vi "COD主界面（列队使用）.vi"() -> (8 "多列列表框":i32(listbox))   [LabVIEW 2016, in "斯坦道CODMn.lvlib"]
uses:
  <vilib>/Utility/miscctls.llb/LVPointTypeDef.ctl
  <vilib>/ptbypt/NI_PtbyPt.lvlib
  <vilib>/Utility/config.llb/NI_LVConfig.lvlib
panel:
  in  "温度补偿":bool
  in  "周期设置":bool
  out "F5":dbl
  out "F4":dbl
  out "F3":dbl
  out "F2":dbl
  out "F1":dbl
  out "F0":dbl
  out "消解压力kPa":dbl format="%#.2f"
  out "权限等级":string
  in  "布尔":bool
  in  "查看曲线":bool
  out "氢氧化钠":dbl
  in  "序列号变更":bool
  out "模块版本号":string
  in  "更新程序":bool
  out "进样无液体告警":bool
  out "60分钟超时报警":bool
  in  "仪器参数":bool
  in  "释放串口":bool
  in  "打开串口":bool
  out "报警数字":i16
  out "CODMn工作状态":T1(ring)
  out "ORP-K":string
  out "ORP-B":string
  out "ORP-A":string
  out "基本量程(显示)":string
  out "测量模式(显示)":string
  out "数据时间":string
  out "断电排液标记":bool
  out "COM":string
  out "空白测试标记":bool
  out "跨度核查标记":bool
  in  "手动控制":bool
  out "启动时间":timestamp format="%<%Y/%m/%d %H:%M:%S>T"
  out "零点核查标记":bool
  out "排液故障":bool
  out "进水样超量程":bool
  out "标样核查标记":bool
  out "平行样测量":bool
  out "加标回收测量":bool
  out "质控样测量":bool
  out "待机":bool
  out "校标错误":bool
  out "校零错误":bool
  out "测量错误":bool
  out "草酸钠报警":bool
  out "高锰酸钾报警":bool
  out "加热故障":bool
  out "温控器故障":bool
  out "ORP故障":bool
  out "排液标记":bool
  out "故障标记":bool
  out "校标标记":bool
  out "校零标记":bool
  out "通讯状态":bool
  out "水样测量":bool
  in  "返回":bool
  in  "校准配置":bool
  out "标度滴定值":dbl
  out "零点滴定值":dbl
  in  "保存":bool
  in  "关闭":bool
  out "仪器时间":timestamp format="%<%Y/%m/%d %H:%M:%S>T"
  out "秒":u16
  out "分":u16
  out "COD浓度（mg/L)":dbl format="%.2g"
  out "进样管":dbl
  out "高锰酸钾":dbl
  out "草酸钠":dbl
  out "硫酸":dbl
  out "实时ORP/光值":dbl
  out "消解温度℃":dbl
  out "加热":bool
  out "搅拌":bool
  out "进硫酸":bool
  out "进加标回收样":bool
  out "进零点核查样":bool
  out "进标液":bool
  out "进蒸馏水":bool
  out "进水样":bool
  out "进草酸钠":bool
  out "进高锰酸钾":bool
  in  "启动":bool
  in  "故障清除":bool
  in  "参数配置":bool
  in  "停止":bool
  in  "单步启动":bool
  out "系统时间":timestamp
  in  "时间校准":bool
  out "模式（受控）":u16
  # "测试时长："
  # "注：遇到加热故障和排液故障时仪器不能正常启动，\n必须排查故障并点击报警清除按钮方可运行。"
  # "mg/L"
  # "校零校标结果"
  # "校零结果："
  # "校零滴定值："
  # "校标结果："
  # "标度滴定值："
  # "零点泵计量值："
  # "标度泵计量值："
  # "校准配置界面"
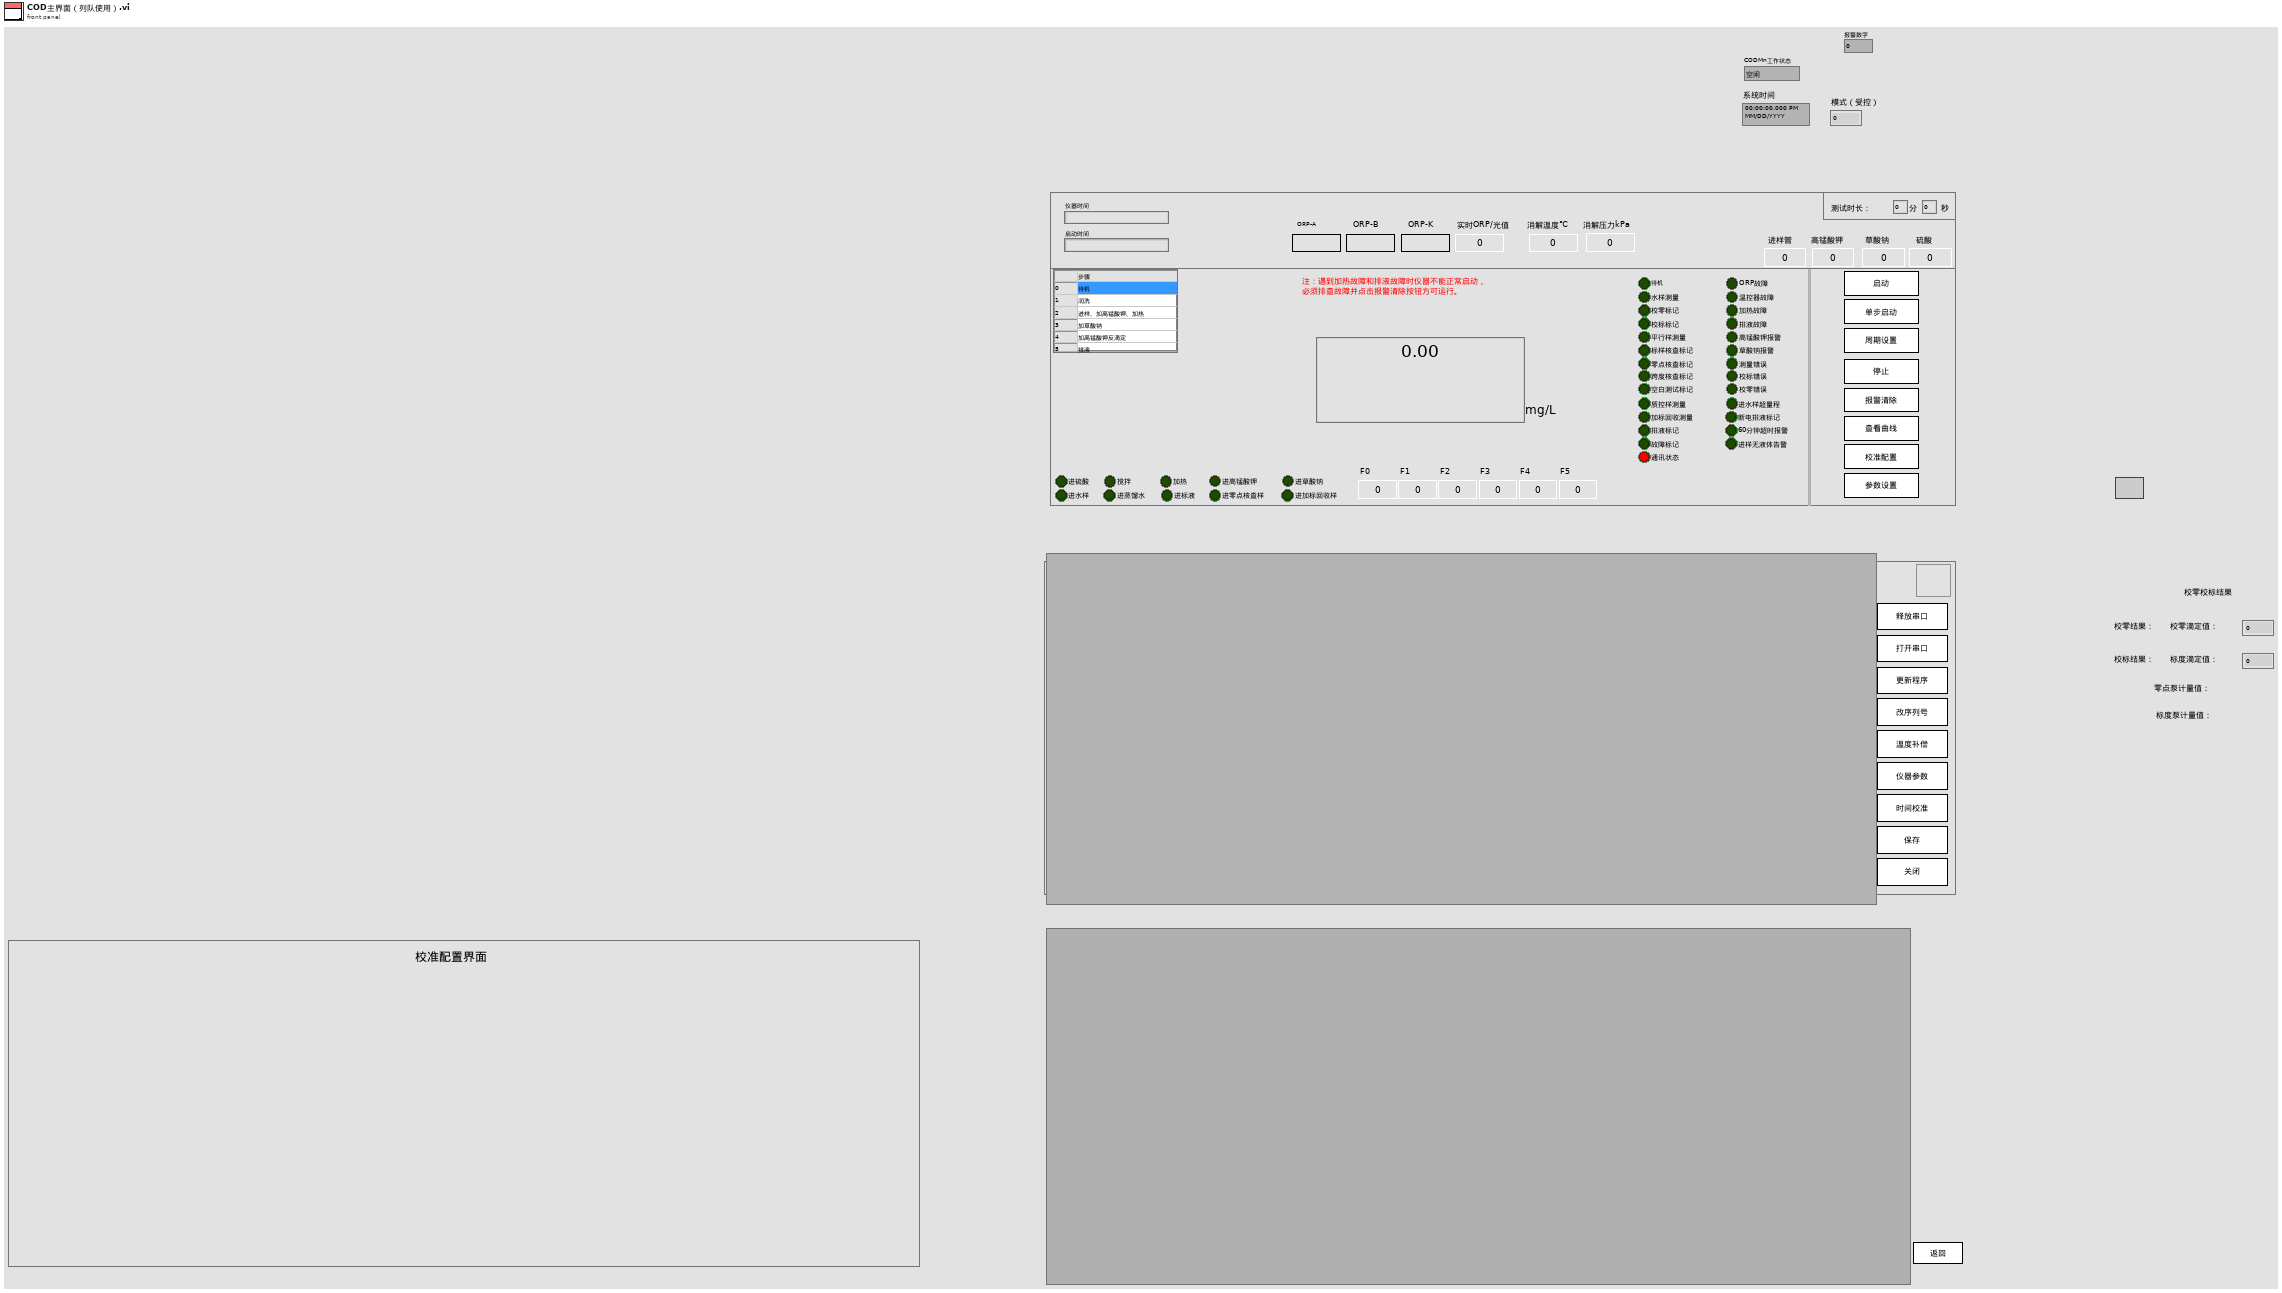
[diagram p1: front panel]
types:
  T1 = enum16{"空闲", "水样测试", "标样核查", "零点核查", "跨度核查", "空白测试", "平行样测试", "质控样", "空白校准", "标样校准", "加标回收"}
  T2 = typedef "LVPointTypeDef.ctl" = cluster{"Horizontal":i16, "Vertical":i16}
  T3 = cluster{"Major":u16, "Minor":u16, "Fix":u16, "Build":u16}
  T4 = typedef "NI_LVConfig.lvlib/Config Data RefNum.ctl" = refnum<k1>
  T5 = cluster{"运行模式":enum16{"维护模式", "常规模式", "应急模式", "质控模式"}, "质控频次":enum16{"关闭", "每天", "星期一", "星期二", "星期三", "星期四", "星期五", "星期六", "星期日"}, "空白核查时间":u16, "跨度核查时间":u16, "测量间隔":u16}
  T6 = cluster{"测量量程":dbl, "测量精度":dbl, "测量间隔":dbl, "消解温度":dbl, "消解时长":dbl, "空白校准时间":timestamp, "曲线截距":dbl, "曲线斜率":dbl, "测量检出限":dbl, "测量信号值":dbl, "线性相关系数":dbl, "二次多项式系数":dbl, "标样校准时间":timestamp, "稀释倍数":dbl, "三项式系数":dbl, "空白标定系数":dbl, "量程系数":dbl, "F0/ORPA":dbl, "F1/ORPB":dbl, "F2/ORPK":dbl, "F3":dbl, "F4":dbl, "F5":dbl, "F6":dbl, "F7":dbl, "X0/滴定数":dbl, "量程":dbl}
  T7 = typedef "TimingControl.lvlib/TimingControl.lvclass/国标控制命令.ctl" = enum16{"启动测量", "标样核查", "零点核查", "跨度核查", "空白测试", "平行样测试", "加标回收", "空白校准", "标样校准", "初始化（清洗）", "停止测试", "仪器重启", "校时", "模式设置", "测量间隔设置"}
  T8 = typedef "TimingControl.lvlib/TimingControl.lvclass/测量参数.ctl" = u16
  T9 = enum32{"Bad", "Idle", "Run top level", "Running"}
  T10 = enum8{"Enabled", "Disabled", "Disabled and Grayed Out"}
  T11 = cluster{"因子编码":u32, "单位":u16, "标样参考值":sgl, "水样数据时间":timestamp, "水样实测值":sgl, "水样数据标识":string, "标样数据时间":timestamp, "标样实测值":sgl, "标样数据标识":string, "空白数据时间":timestamp, "空白实测值":sgl, "空白数据标识":string, "零点核查数据时间":timestamp, "零点核查实测值":sgl, "零点核查数据标识":string, "跨度核查数据时间":timestamp, "跨度核查实测值":sgl, "跨度核查数据标识":string, "加标回收数据时间":timestamp, "加标回收实测值":sgl, "加标回收数据标识":string, "平行样数据时间":timestamp, "平行样实测值":sgl, "平行样数据标识":string}
  T12 = cluster{"时间":timestamp, "测量模式":string, "数据类型":string, "检测值":sgl, "单位":string, "数据标识":string, "因子编码":string, "标样参考值":sgl, "ORP-A":sgl, "ORP-B":sgl, "ORP-K":sgl, "COD滴定值":sgl, "高锰酸钾滴定数":sgl, "温度":sgl, "量程":sgl, "LastTime":timestamp, "序列号:":string, "跨度值":sgl, "高锰酸钾原始滴定数":sgl, "F0":sgl, "F1":sgl, "F2":sgl, "F3":sgl, "F4":sgl, "F5":sgl}
  T13 = cluster{"ORP故障":bool, "温控器故障":bool, "加热故障":bool, "高锰酸钾报警":bool, "草酸钠报警":bool, "测量错误":bool, "校零错误":bool, "校标错误":bool, " 进水样超量程":bool, "排液阀故障":bool, "60分钟超时报警":bool, "进样无液体报警":bool}
  T14 = cluster{"时间":timestamp, "水样计量数":u16, "蒸馏水计量数":u16, "标液计量数":u16, "零点核查计量数":u16, "加标回收计量数":u16, "硫酸计量数":u16, "高锰酸钾计量数":u16, "草酸钠计量数":u16, "更换泵管":string}
  T15 = cluster{"确定":bool, "测量量程":dbl, "测量精度":dbl, "测量间隔":dbl, "消解温度":dbl, "消解时长":dbl, "空白校准时间":timestamp, "曲线截距":dbl, "曲线斜率":dbl, "测量检出限":dbl, "测量信号值":dbl, "线性相关系数":dbl, "二次多项式系数":dbl, "标样校准时间":timestamp, "稀释倍数":dbl, "三项式系数":dbl, "空白标定系数":dbl, "量程系数":dbl, "F0/ORPA":dbl, "F1/ORPB":dbl, "F2/ORPK":dbl, "F3":dbl, "F4":dbl, "F5":dbl, "F6":dbl, "F7":dbl, "X0/滴定数":dbl, "量程":dbl}
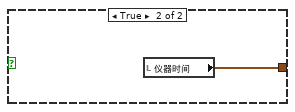
[diagram p6: hidden frame]
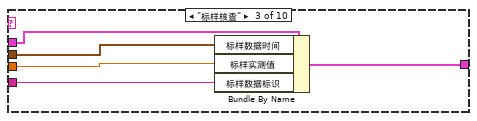
[diagram p13: hidden frame]
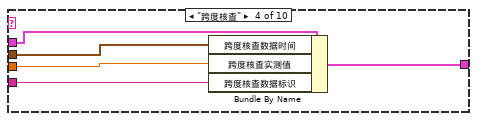
[diagram p14: hidden frame]
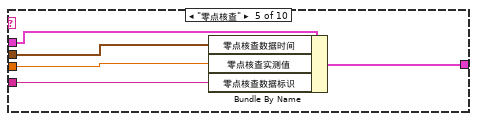
[diagram p15: hidden frame]
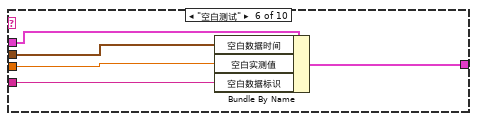
[diagram p16: hidden frame]
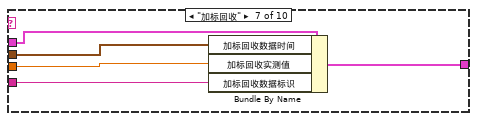
[diagram p17: hidden frame]
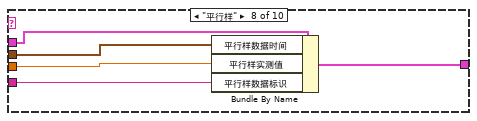
[diagram p18: hidden frame]
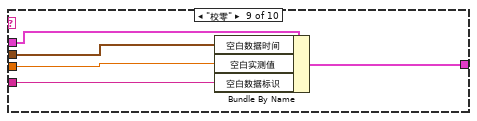
[diagram p19: hidden frame]
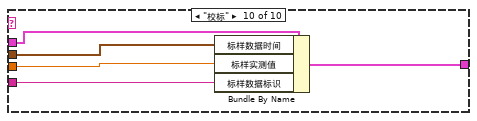
[diagram p20: hidden frame]
diagram:
  n1 = control-ref of="周期设置"() -> (w5:refnum<vi>)
  n2 = call "New TimingControl.vi"("Reference"=w5) -> ("error out"=w3:errorcluster, "TimingControl out"=w4:refnum<class "TimingControl.lvclass">)  [unwired: 9 in]
  n3 = call "taskqueue ref.vi"() -> ("队列输出"=w16:refnum<queue>)  [unwired: 10 in, 1 out]
  n4 = call "task.vi"() -> ()  [unwired: 12 in]
  n5 = flat-sequence {
    tunnel: [w33] -> w19
    tunnel: [errorcluster {"status"=FALSE, "code"=0, "source"=""} ("错误输出")] -> w17
    tunnel: [w35] -> w18
    frame #0 {
      w57 = "192.168.1.100" ("名称")
      n6 = global read "COD内部交互全局.vi" "序列号:"() -> (w64:string)
      n7 = global write "COD内部交互全局.vi" "量程切换次数"(u8 0 ("量程切换次数")) -> ()
      n8 = global write "COD内部交互全局.vi" "切换量程连续测两次"(FALSE ("切换量程连续测两次")) -> ()
      n9 = property on="窗格" class="Pane"("Origin"=T2 {"Horizontal"=0, "Vertical"=0} ("原点")) -> ()  [unwired: 2 in, 2 out]
      n10 = control-ref of="本VI"() -> (w44:refnum<vi>)
      n11 = property class="VI"(reference=w44) -> ("Library.Version"=w43:T3)  [unwired: 1 in, 2 out]
      n12 = Empty String/Path?(string/path=w64) -> (empty?=w32:bool)
      n13 = case shown="真" w32 {
        tunnel: w64 -> [w76 _]
        tunnel: [w75 "data\\CODMnSet.ini" ("名称或相对路径")] -> w45
        frame False {
          # "与生产用上位机交互"
          n14 = Concatenate Strings("data\\" ("字符串"), "序列号" ("字符串"), w76, "Set.ini" ("名称或相对路径")) -> (w75:string)
        }
        frame True {
        }
      }
      n15 = Unbundle By Name(w43) -> ("Major"=w41:u16, "Minor"=w40:u16, "Fix"=w39:u16, "Build"=w38:u16)
      n16 = String To IP(1:w57) -> (0:w50:u32)
      n17 = Format Into String(format string="模块版本号：%d.%d.%d.%d" ("格式字符串"), w41, w40, w39, w38) -> (resulting string=→"模块版本号":string)  [unwired: 2 in, 1 out]
      n18 = IP To String(2:w50) -> (0:w53:string)  [unwired: 1 in]
      n19 = Not Equal?(x=w57, y=w53) -> (x != y?=w58:bool)
      n20 = Concatenate Strings("\\\\" ("字符串"), w53) -> (w52:string)
      n21 = global write "CODMN外部API.vi" "ping"(w58) -> ()
      n22 = String To Path(string=w52) -> (path=w59:path)
      n23 = global write "COD内部交互全局.vi" "配置文件ini"(w45) -> ()
      n24 = Build Path(base path=w59, name or relative path=w45) -> (appended path=w54:path)
      n25 = case shown="真" w58 {
        tunnel: w54 -> [w66 w70]
        tunnel: [w66 w69] -> w55
        tunnel: [FALSE w68] -> w56
        frame False {
        }
        frame True {
          n26 = call <vilib>:"Check if File or Folder Exists.vi"("path"=w70) -> ("file or folder exists?"=w68:bool, "dup path"=w69:path)  [unwired: 8 in, 1 out]
        }
      }
      n27 = case shown="假" w56 {
        tunnel: w55 -> [_ w74]
        tunnel: [w72 w74] -> w36
        tunnel: w45 -> [w71 _]
        frame False {
          # "本地文件地址"
          n28 = call <vilib>:"Application Directory.vi"() -> ("Application Directory"=w73:path)
          n29 = Build Path(base path=w73, name or relative path=w71) -> (appended path=w72:path)
        }
        frame True {
          # "网络共享地址"
        }
      }
      n30 = global write "CODMN外部API.vi" "配置文件 path"(w36) -> ()
      n31 = call <vilib>:"Open Config Data.vi"("configuration file path"=w36) -> ("error out"=w46:errorcluster, "refnum"=w47:T4)  [unwired: 8 in, 1 out]
      n32 = vi-ref "斯坦道CODMn.lvlib:CODMn断电保存全局变量.vi"() -> (w60:refnum<vi>)
      n33 = call <userlib>:"Read Panel from INI__ogtk.vi"("error in (no error)"=w46, "VI ref"=w60, "refnum"=w47) -> ("error out"=w48:errorcluster, "refnum out"=w49:T4)  [unwired: 7 in]
      n34 = call <vilib>:"Close Config Data.vi"("error in (no error)"=w48, "refnum"=w49) -> ("error out"=w34:errorcluster)  [unwired: 8 in, 1 out]
      n35 = call <vilib>:"Clear Errors.vi"("error in (no error)"=w34) -> ("error out"=w31:errorcluster)  [unwired: 5 in, 1 out]
      n36 = Read from Text File(file (use dialog)=w36, error in=w31) -> (text=w35:string, error out=w33:errorcluster)  [unwired: 2 in, 2 out]
    }
  }
  n37 = while {
    stop <- FALSE stop-if-true
    # "相差60秒自动校时"
    n38 = global read "运行时序全局变量.vi" "多列列表框"() -> (w84:i32)
    n39 = local read "消解温度℃"() -> (w81:dbl)
    n40 = local read "仪器时间"() -> (w91:timestamp)
    n41 = local read "系统时间"() -> (w92:timestamp)
    n42 = Wait (ms)(milliseconds to wait=u32 1000 ("等待时间（毫秒）")) -> ()  [unwired: 1 out]
    n43 = call "消解压力计算.vi"("当前消解温度"=w81) -> ("消解压力"=→"消解压力kPa":dbl)  [unwired: 10 in]
    n44 = Build Array(w91) -> (w90:timestamp[])
    n45 = Build Array(w92) -> (w109:timestamp[])
    n46 = Equal?(x=w84, y=u16 5) -> (x = y?=w86:bool)
    n47 = call <vilib>:"Boolean Crossing PtByPt.vi"("direction"=enum16{"either", "false-true", "true-false"}."false-true", "input"=w86) -> ("crossing"=w83:bool)  [unwired: 1 in]
    n48 = call "DateToHex.vi"("DATE"=w90) -> ("数组"=w103:u16[])  [unwired: 10 in]
    n49 = call "DateToHex.vi"("DATE"=w109) -> ("数组"=w108:u16[])  [unwired: 10 in]
    n50 = case shown="真" w83 {
      frame False {
      }
      frame True {
        # "校准结束后自动更新曲线泵滴定数"
        n51 = global read "CODMN外部API.vi" "远程反控校准CODMn"() -> (w110:bool)
        n52 = case shown="真" w110 {
          frame False {
          }
          frame True {
            # "校准完自动写入公式"
            n53 = global write "CODMN外部API.vi" "远程反控校准CODMn"(FALSE ("远程反控校准CODMn")) -> ()
          }
        }
      }
    }
    n54 = Index Array(array=w103, index=2 ("索引")) -> (element=w105:u16)
    n55 = Index Array(array=w108, index=2 ("索引")) -> (element=w106:u16)
    n56 = Split Number(x=w105) -> (hi(x)=w99:u8)  [unwired: 1 out]
    n57 = Split Number(x=w106) -> (hi(x)=w102:u8)  [unwired: 1 out]
    n58 = To Byte Integer(number=w99) -> (8bit integer=w98:i8)
    n59 = To Byte Integer(number=w102) -> (8bit integer=w101:i8)
    n60 = Subtract(x=w98, y=w101) -> (x-y=w100:i8)
    n61 = Absolute Value(x=w100) -> (abs(x)=w97:i8)
    n62 = local read "通讯状态"() -> (w94:bool)
    n63 = Greater Or Equal?(x=w97, y=i8 5) -> (x >= y?=w95:bool)
    n64 = And(x=w95, y=w94) -> (x .and. y?=w93:bool)
    n65 = case shown="真" w93 {
      frame False {
      }
      frame True {
        # "相差60秒时间自动校准"
        n66 = flat-sequence {
          frame #0 {
            n67 = property on="时间校准" class="Bool (严格)"("Val(Sgnl)"=TRUE ("值(信号)")) -> ()  [unwired: 2 in, 2 out]
          }
          frame #1 {
            n68 = Wait (ms)(milliseconds to wait=u32 500 ("等待时间（毫秒）")) -> ()  [unwired: 1 out]
          }
          frame #2 {
            n69 = property on="时间校准" class="Bool (严格)"("Val(Sgnl)"=FALSE ("值(信号)")) -> ()  [unwired: 2 in, 2 out]
          }
        }
      }
    }
  }
  n70 = while {
    tunnel: w16 -> [w133]
    shift-right: [w125] -> _
    shift-left: 0 -> [w124]
    shift-right: [w116] -> w2
    shift-left: w4 -> [w121]
    shift-right: [w115] -> w1
    shift-left: w3 -> [w120]
    stop <- FALSE stop-if-true
    n71 = global read "CODMn断电保存全局变量.vi" "运行周期"() -> (w135:T5)
    n72 = local read "通讯状态"() -> (w138:bool)
    n73 = Quotient & Remainder(x=w124, y=30) -> (x-y*floor(x/y)=w122:i32)  [unwired: 1 out]
    n74 = Equal To 0?(x=w122) -> (x = 0?=w129:bool)
    n75 = global read "CODMn断电保存全局变量.vi" "CODMn仪器参数"() -> (w137:T6)
    n76 = Unbundle By Name(w135) -> ("测量间隔"=w134:u16)
    n77 = case shown="假" w138 {
      tunnel: [w149 w150] -> w118
      frame False {
        n78 = Get Date/Time In Seconds() -> (seconds since 1Jan1904=w149:timestamp)
      }
      frame True {
        n79 = local read "仪器时间"() -> (w150:timestamp)
      }
    }
    n80 = Bundle By Name(cluster=w137, "测量间隔"=w134) -> (w136:T6)
    n81 = global read "COD测量模式全局.vi" "CODMn工作状态"() -> (w130:T1)
    n82 = Not Equal?(x=w130, y=T1."空闲") -> (x != y?=w117:bool)
    n83 = global write "CODMn断电保存全局变量.vi" "CODMn仪器参数"(w136) -> ()
    n84 = property class="TimingControl"(reference=w121, error in=w120, "Properties:仪器时间"=w118, "Properties:仪器运行状态"=w117) -> (reference out=w116:refnum<class "TimingControl.lvclass">, error out=w115:errorcluster, "Properties:命令输出"=w119:cluster{"启动":bool, "控制命令":T7, "测量参数":T8})
    n85 = Increment(x=w124) -> (x+1=w127:i32)
    n86 = Unbundle By Name(w119) -> ("启动"=w128:bool, "控制命令"=w132:T7)
    n87 = And(x=w128, y=w129) -> (x .and. y?=w131:bool)
    n88 = Select(t=w127, s=w128, f=0) -> (s? t:f=w125:i32)
    n89 = case shown="真" w131 {
      tunnel: w133 -> [_ w146]
      tunnel: w132 -> [_ w145]
      frame False {
      }
      frame True {
        n90 = Get Queue Status(queue=w146) -> (queue out=w144:refnum<queue>, # elements in queue=w143:i32)  [unwired: 2 in, 6 out]
        n91 = Equal To 0?(x=w143) -> (x = 0?=w142:bool)
        n92 = case shown="真" w142 {
          tunnel: w145 -> [_ w148]
          tunnel: w144 -> [_ w147]
          frame False {
          }
          frame True {
            n93 = Enqueue Element(queue=w147, element=w148) -> ()  [unwired: 2 in, 3 out]
          }
        }
      }
    }
    n94 = Wait (ms)(milliseconds to wait=u32 500 ("等待时间（毫秒）")) -> ()  [unwired: 1 out]
  }
  n95 = vi-ref "斯坦道CODMn.lvlib:参数设置页.vi"() -> (w7:refnum<vi>)
  n96 = vi-ref "校准设置页.vi"() -> (w14:refnum<vi>)
  n97 = property class="VI"(reference=w7) -> (reference out=w9:refnum<vi>, "Exec.State"=w8:T9)  [unwired: 1 in, 1 out]
  n98 = property class="VI"(reference=w14) -> (reference out=w12:refnum<vi>, "Exec.State"=w13:T9)  [unwired: 1 in, 1 out]
  n99 = case shown="\"Idle\"" w8 {
    tunnel: w9 -> [w151 w155]
    tunnel: [w151 w152] -> w6
    frame "Bad", Default {
    }
    frame "Idle" {
      n100 = invoke class="VI" method="Run VI"(reference=w155, "Wait until done"=FALSE ("结束前等待"), "Auto Dispose Ref"=TRUE ("自动销毁引用")) -> (reference out=w152:refnum<vi>)  [unwired: 2 in, 4 out]
    }
  }
  n101 = case shown="\"Idle\"" w13 {
    tunnel: w12 -> [w156 w160]
    tunnel: [w156 w157] -> w11
    frame "Bad", Default {
    }
    frame "Idle" {
      n102 = invoke class="VI" method="Run VI"(reference=w160, "Wait until done"=FALSE ("结束前等待"), "Auto Dispose Ref"=TRUE ("自动销毁引用")) -> (reference out=w157:refnum<vi>)  [unwired: 2 in, 4 out]
    }
  }
  n103 = call "Close TimingControl.vi"("error in (no error)"=w1, "TimingControl in"=w2) -> ()  [unwired: 9 in, 1 out]
  n104 = Obtain Queue(name (unnamed)="CODMn", element data type=cluster{"命令":string} {"命令"="启用模块"} ("元素")) -> (queue out=w29:refnum<queue>, error out=w28:errorcluster)  [unwired: 3 in, 1 out]
  n105 = while {
    tunnel: w19 -> [_]
    stop <- FALSE stop-if-true
    # "赋值循环"
    n106 = flat-sequence {
      frame #0 {
        # "局部变量给内部交互用全局变量"
        n107 = local read "待机"() -> (w168:bool)
        n108 = local read "实时ORP/光值"() -> (w163:dbl)
        n109 = local read "消解温度℃"() -> (w164:dbl)
        n110 = local read "多列列表框"() -> (w170:i32)
        n111 = local read "故障标记"() -> (w171:bool)
        n112 = local read "高锰酸钾"() -> (w165:dbl)
        n113 = global write "COD内部交互全局.vi" "待机"(w168) -> ()
        n114 = local read "COD浓度（mg/L)"() -> (w169:dbl)
        n115 = local read "CODMn工作状态"() -> (w172:T1)
        n116 = local read "断电排液标记"() -> (w166:bool)
        n117 = local read "高锰酸钾报警"() -> (w167:bool)
        n118 = global write "COD内部交互全局.vi" "故障标记"(w171) -> ()
        n119 = global write "COD内部交互全局.vi" "ORP显示"(w163) -> ()
        n120 = global write "COD内部交互全局.vi" "高锰酸钾"(w165) -> ()
        n121 = global write "COD内部交互全局.vi" "实时温度"(w164) -> ()
        n122 = global write "运行时序全局变量.vi" "多列列表框"(w170) -> ()
        n123 = global write "COD浓度全局变量.vi" "COD浓度（mg/L)"(w169) -> ()
        n124 = global write "COD内部交互全局.vi" "断电排液标记"(w166) -> ()
        n125 = global write "COD内部交互全局.vi" "高锰酸钾报警"(w167) -> ()
        n126 = global write "COD测量模式全局.vi" "CODMn工作状态"(w172) -> ()
      }
    }
    n127 = flat-sequence {
      frame #0 {
        # "断电保存全局给局部变量"
        n128 = global read "CODMn断电保存全局变量.vi" "启动时间"() -> (→"启动时间":timestamp)
      }
    }
    n129 = flat-sequence {
      frame #0 {
        # "显示量程说明"
        n130 = global read "COD内部交互全局.vi" "通讯状态"() -> (→"通讯状态":bool)
        n131 = global read "CODMn断电保存全局变量.vi" "MB通信方式选择"() -> (w238:enum16{"串口", "TCP"})
        n132 = case shown="\"TCP\"" w238 {
          tunnel: [w241 w242] -> w240
          frame "串口", Default {
            n133 = global read "CODMn断电保存全局变量.vi" "VISA resource name"() -> (w241:refnum<visa-resource-name>)
          }
          frame "TCP" {
            n134 = global read "CODMn断电保存全局变量.vi" "IP"() -> (w242:string)
          }
        }
        "COM" <- w240
      }
    }
    n135 = flat-sequence {
      frame #0 {
        # "权限隐藏和显示功能"
        n136 = global read "CODMN外部API.vi" "权限等级"() -> (w248:enum16{"一级权限", "二级权限", "三级权限", "超级权限"})
        n137 = global read "CODMn断电保存全局变量.vi" "常规版/认证版"() -> (w244:enum16{"常规版-酸性", "常规版-碱性", "认证版", "浮台版"})
        n138 = case shown="\"二级权限\"" w248 {
          tunnel: [w253 FALSE w258 w260] -> w245
          tunnel: ["一级权限" "二级权限" "三级权限" "超级权限"] -> w247
          tunnel: [w253 TRUE w258 w260] -> w246
          frame "一级权限", Default {
            w253 = FALSE
          }
          frame "二级权限" {
          }
          frame "三级权限" {
            w258 = TRUE
          }
          frame "超级权限" {
            w260 = TRUE
          }
        }
        "权限等级" <- w247
        n139 = global read "CODMn断电保存全局变量.vi" "CODMn系统周期测试?"() -> (w249:bool)
        n140 = case shown="\"浮台版\"" w244 {
          tunnel: [T10."Enabled" ("禁用") T10."Enabled" ("禁用") T10."Disabled and Grayed Out" ("禁用") T10."Enabled" ("禁用")] -> _
          tunnel: [i32[] [2] ("禁用项[]") i32[] [2] ("禁用项[]") i32[] [] ("禁用项[]") i32[] [2] ("禁用项[]")] -> _
          tunnel: [w271 w276 T10."Disabled and Grayed Out" ("禁用") w287] -> _
          tunnel: [w270 FALSE FALSE TRUE] -> _
          tunnel: [w271 w276 T10."Disabled and Grayed Out" ("禁用") w287] -> w252
          tunnel: [w270 TRUE FALSE FALSE] -> w251
          frame "常规版-酸性", Default {
            w270 = FALSE
            w271 = T10."Enabled" ("禁用")
          }
          frame "常规版-碱性" {
            w276 = T10."Enabled" ("禁用")
          }
          frame "认证版" {
            w282 = u16 1 items=["水样测试"=1, "标样核查"=2, "零点核查"=3, "跨度核查"=4, "空白测试"=5, "平行样"=6, "加标回收"=7] ("测量模式(公式)")
            n141 = global write "CODMn断电保存全局变量.vi" "测量模式(公式)"(w282) -> ()
          }
          frame "浮台版" {
            w287 = T10."Enabled" ("禁用")
          }
        }
        n142 = global read "CODMn断电保存全局变量.vi" "运行周期"() -> (w250:T5)
        n143 = case shown="真" w249 {
          tunnel: w250 -> [_ w265]
          tunnel: [T10."Enabled" ("禁用") w263] -> _
          frame False {
          }
          frame True {
            n144 = Unbundle By Name(w265) -> ("运行模式"=w264:enum16{"维护模式", "常规模式", "应急模式", "质控模式"})
            n145 = case shown="\"维护模式\", 默认" w264 {
              tunnel: [T10."Enabled" ("禁用") T10."Disabled and Grayed Out" ("禁用") T10."Disabled and Grayed Out" ("禁用") T10."Disabled and Grayed Out" ("禁用")] -> w263
              frame "维护模式", Default {
              }
              frame "常规模式" {
              }
              frame "应急模式" {
              }
              frame "质控模式" {
              }
            }
          }
        }
        n146 = property on="更新程序" class="Bool (严格)"("Visible"=w245) -> ()  [unwired: 2 in, 2 out]
        n147 = property on="释放串口" class="Bool"("Visible"=w246) -> ()  [unwired: 2 in, 2 out]
        n148 = property on="打开串口" class="Bool"("Visible"=w246) -> ()  [unwired: 2 in, 2 out]
        n149 = property on="序列号变更" class="Bool"("Visible"=w245) -> ()  [unwired: 2 in, 2 out]
        n150 = property on="氢氧化钠" class="DigNum (严格)"("Visible"=w251) -> ()  [unwired: 2 in, 2 out]
        n151 = control-ref of="进样管"() -> (w243:refnum<vi>)
        n152 = property class="DigNum (严格)"(reference=w243, "DisabledEnum"=w252) -> ()  [unwired: 1 in, 2 out]
      }
    }
    n153 = flat-sequence {
      frame #0 {
        # "测量数据区"
        n154 = global read "CODMn断电保存全局变量.vi" "测量数据区"() -> (w185:T11)
        n155 = global read "COD内部交互全局.vi" "data"() -> (w190:T12)
        n156 = global read "COD测量模式全局.vi" "测量模式文字实时"() -> (w176:string)
        "测量模式(显示)" <- w176
        n157 = global read "CODMn断电保存全局变量.vi" "水样测试量程"() -> (w178:enum16{"L", "H"})
        n158 = Unbundle By Name(w185) -> ("水样实测值"=w182:sgl)
        n159 = global read "CODMn断电保存全局变量.vi" "测量模式"() -> (w174:string)
        n160 = Unbundle By Name(w190) -> ("时间"=w189:timestamp, "检测值"=w188:sgl, "数据标识"=w187:string)
        n161 = feedback-in #1(w185) -> ()
        n162 = feedback #1(w185) -> (w184:T11)
        n163 = Unbundle By Name(w184) -> ("水样实测值"=w183:sgl)
        n164 = case shown="\"水样测试\"" w176 {
          tunnel: w185 -> [w191 w196 w201 w206 w211 w216 w221 w226 w231 w236]
          tunnel: [w191 w195 w200 w202 w210 w215 w220 w225 w227 w235] -> w186
          tunnel: w189 -> [_ w194 w199 w205 w209 w214 w219 w224 w230 w234]
          tunnel: w188 -> [_ w193 w198 w204 w208 w213 w218 w223 w229 w233]
          tunnel: w187 -> [_ w192 w197 w203 w207 w212 w217 w222 w228 w232]
          frame "", Default {
          }
          frame "水样测试" {
            n165 = Bundle By Name(cluster=w196, "水样数据时间"=w194, "水样实测值"=w193, "水样数据标识"=w192) -> (w195:T11)
          }
          frame "标样核查" {
            n166 = Bundle By Name(cluster=w201, "标样数据时间"=w199, "标样实测值"=w198, "标样数据标识"=w197) -> (w200:T11)
          }
          frame "跨度核查" {
            n167 = Bundle By Name(cluster=w206, "跨度核查数据时间"=w205, "跨度核查实测值"=w204, "跨度核查数据标识"=w203) -> (w202:T11)
          }
          frame "零点核查" {
            n168 = Bundle By Name(cluster=w211, "零点核查数据时间"=w209, "零点核查实测值"=w208, "零点核查数据标识"=w207) -> (w210:T11)
          }
          frame "空白测试" {
            n169 = Bundle By Name(cluster=w216, "空白数据时间"=w214, "空白实测值"=w213, "空白数据标识"=w212) -> (w215:T11)
          }
          frame "加标回收" {
            n170 = Bundle By Name(cluster=w221, "加标回收数据时间"=w219, "加标回收实测值"=w218, "加标回收数据标识"=w217) -> (w220:T11)
          }
          frame "平行样" {
            n171 = Bundle By Name(cluster=w226, "平行样数据时间"=w224, "平行样实测值"=w223, "平行样数据标识"=w222) -> (w225:T11)
          }
          frame "校零" {
            n172 = Bundle By Name(cluster=w231, "空白数据时间"=w230, "空白实测值"=w229, "空白数据标识"=w228) -> (w227:T11)
          }
          frame "校标" {
            n173 = Bundle By Name(cluster=w236, "标样数据时间"=w234, "标样实测值"=w233, "标样数据标识"=w232) -> (w235:T11)
          }
        }
        n174 = feedback #2(w178) -> (w179:enum16{"L", "H"})
        n175 = feedback-in #2(w178) -> ()
        n176 = feedback #3(w174) -> (w175:string)
        n177 = feedback-in #3(w174) -> ()
        n178 = Not Equal?(x=w175, y=w174) -> (x != y?=w173:bool)
        n179 = Not Equal?(x=w179, y=w178) -> (x != y?=w177:bool)
        n180 = Not Equal?(x=w182, y=w183) -> (x != y?=w181:bool)
        n181 = Compound Arithmetic op=OR ("复合运算")(w181, w177, w173) -> (w180:bool)
        n182 = case shown="真" w180 {
          frame False {
          }
          frame True {
            # "水样值发送改变存储本地"
            n183 = call "配置文件保存.vi"() -> ()  [unwired: 12 in]
          }
        }
        n184 = global write "CODMn断电保存全局变量.vi" "测量数据区"(w186) -> ()
      }
    }
    n185 = Wait (ms)(milliseconds to wait=u32 1000 ("等待时间（毫秒）")) -> ()  [unwired: 1 out]
  }
  n186 = while {
    tunnel: [w297] -> _
    shift-right: [w295] -> _
    shift-left: w18 -> [w294]
    tunnel: w19 -> [_]
    stop <- FALSE stop-if-true
    n187 = Wait (ms)(milliseconds to wait=u32 1000 ("等待时间（毫秒）")) -> ()  [unwired: 1 out]
    n188 = global read "CODMN外部API.vi" "配置文件 path"() -> (w291:path)
    n189 = Read from Text File(file (use dialog)=w291) -> (text=w295:string, error out=w292:errorcluster)  [unwired: 3 in, 2 out]
    n190 = Not Equal?(x=w295, y=w294) -> (x != y?=w293:bool)
    n191 = case shown="真" w293 {
      tunnel: [w299 w306] -> w297
      tunnel: w291 -> [_ w300]
      tunnel: w292 -> [w299 _]
      frame False {
      }
      frame True {
        # "文件发生改变进行更新，远端和本地都更新"
        n192 = call <vilib>:"Open Config Data.vi"("configuration file path"=w300) -> ("error out"=w305:errorcluster, "refnum"=w304:T4)  [unwired: 8 in, 1 out]
        n193 = vi-ref "斯坦道CODMn.lvlib:CODMn断电保存全局变量.vi"() -> (w301:refnum<vi>)
        n194 = call <userlib>:"Read Panel from INI__ogtk.vi"("error in (no error)"=w305, "VI ref"=w301, "refnum"=w304) -> ("error out"=w303:errorcluster, "refnum out"=w302:T4)  [unwired: 7 in]
        n195 = call <vilib>:"Close Config Data.vi"("error in (no error)"=w303, "refnum"=w302) -> ("error out"=w306:errorcluster)  [unwired: 8 in, 1 out]
      }
    }
  }
  n196 = flat-sequence {
    tunnel: w17 -> [_]
    frame #0 {
      n197 = vi-ref "斯坦道CODMn.lvlib:关键参数交互.vi"() -> (w324:refnum<vi>)
      n198 = vi-ref "斯坦道CODMn.lvlib:时间-温度曲线(子VI).vi"() -> (w315:refnum<vi>)
      n199 = property class="VI"(reference=w324, error in=errorcluster {"status"=FALSE, "code"=0, "source"=""} ("错误输出")) -> ("Name"=w323:string)  [unwired: 2 out]
      n200 = vi-ref "斯坦道CODMn.lvlib:高锰酸钾-ORP滴定曲线(子VI).vi"() -> (w333:refnum<vi>)
      n201 = vi-ref "斯坦道CODMn.lvlib:日志报警状态存储 (子VI).vi"() -> (w346:refnum<vi>)
      n202 = vi-ref "斯坦道CODMn.lvlib:待机状态数据存储写入和切换量程(子VI).vi"() -> (w353:refnum<vi>)
      n203 = property class="VI"(reference=w315, error in=errorcluster {"status"=FALSE, "code"=0, "source"=""} ("错误输出")) -> ("Name"=w314:string)  [unwired: 2 out]
      n204 = property class="VI"(reference=w346, error in=errorcluster {"status"=FALSE, "code"=0, "source"=""} ("错误输出")) -> ("Name"=w345:string)  [unwired: 2 out]
      n205 = property class="VI"(reference=w333, error in=errorcluster {"status"=FALSE, "code"=0, "source"=""} ("错误输出")) -> ("Name"=w334:string)  [unwired: 2 out]
      n206 = Open VI Reference(type specifier VI Refnum (for type only)=refnum<vi> refnum, vi path=w323, options=128 ("选项")) -> (vi reference=w325:refnum<vi>, error out=w321:errorcluster)  [unwired: 3 in]
      n207 = property class="VI"(reference=w353, error in=errorcluster {"status"=FALSE, "code"=0, "source"=""} ("错误输出")) -> ("Name"=w352:string)  [unwired: 2 out]
      n208 = Open VI Reference(type specifier VI Refnum (for type only)=refnum<vi> refnum, vi path=w314, options=128 ("选项")) -> (vi reference=w316:refnum<vi>, error out=w312:errorcluster)  [unwired: 3 in]
      n209 = Open VI Reference(type specifier VI Refnum (for type only)=refnum<vi> refnum, vi path=w345, options=128 ("选项")) -> (vi reference=w329:refnum<vi>, error out=w343:errorcluster)  [unwired: 3 in]
      n210 = Open VI Reference(type specifier VI Refnum (for type only)=refnum<vi> refnum, vi path=w334, options=128 ("选项")) -> (vi reference=w332:refnum<vi>, error out=w336:errorcluster)  [unwired: 3 in]
      n211 = call-by-ref "?"(reference=w316, error in=w312) -> (reference out=w310:refnum<vi>, error out=w311:errorcluster)  [unwired: 12 in]
      n212 = call-by-ref "?"(reference=w325, error in=w321, "量程选择"=enum16{"低量程", "高量程"}."低量程", "模型"=enum32{"线性", "多项式", "折线"}."线性") -> (reference out=w319:refnum<vi>, error out=w320:errorcluster)  [unwired: 10 in]
      n213 = Close Reference(reference=w310, error in (no error)=w311) -> ()  [unwired: 1 out]
      n214 = Close Reference(reference=w319, error in (no error)=w320) -> ()  [unwired: 1 out]
      n215 = call-by-ref "?"(reference=w329, error in=w343) -> (reference out=w341:refnum<vi>, error out=w342:errorcluster)  [unwired: 12 in]
      n216 = call-by-ref "?"(reference=w332, error in=w336) -> (reference out=w338:refnum<vi>, error out=w337:errorcluster)  [unwired: 12 in]
      n217 = Open VI Reference(type specifier VI Refnum (for type only)=refnum<vi> refnum, vi path=w352, options=128 ("选项")) -> (vi reference=w327:refnum<vi>, error out=w350:errorcluster)  [unwired: 3 in]
      n218 = Close Reference(reference=w341, error in (no error)=w342) -> ()  [unwired: 1 out]
      n219 = Close Reference(reference=w338, error in (no error)=w337) -> ()  [unwired: 1 out]
      n220 = call-by-ref "?"(reference=w327, error in=w350) -> (reference out=w348:refnum<vi>, error out=w349:errorcluster)  [unwired: 12 in]
      n221 = Close Reference(reference=w348, error in (no error)=w349) -> ()  [unwired: 1 out]
    }
  }
  n222 = vi-ref "CODMn通讯.vi"() -> (w20:refnum<vi>)
  n223 = while {
    tunnel: w29 -> [w363]
    tunnel: w28 -> [w362]
    tunnel: w19 -> [_]
    stop <- FALSE stop-if-true
    # "主循环界面显示"
    n224 = flat-sequence {
      frame #0 {
        # "A，B，K"
        # "CODMn读取状态"
        n225 = global read "COD内部交互全局.vi" "ORP、时间"() -> (w510:u16[])
        n226 = To Word Integer(number=w510) -> (16bit integer=w528:i16[])
        n227 = Split 1D Array(array=w528, index=3 ("索引")) -> (first subarray=w512:i16[], second subarray=w527:i16[])
        n228 = global read "CODMn断电保存全局变量.vi" "屏蔽负值"() -> (w508:bool)
        n229 = Index Array(array=w512) -> (element #1=w516:i16, element #2=w515:i16, element #3=w514:i16)  [unwired: 3 in]
        n230 = Index Array(array=w527) -> (element #1=w507:i16, element #2=w526:i16, element #3=w525:i16, element #4=w524:i16)  [unwired: 4 in]
        n231 = case shown="真" w508 {
          selector: w508 -> [w530 _]
          tunnel: w507 -> [w532 w537]
          tunnel: [w531 w540] -> w506
          tunnel: [w530 w536] -> _
          frame False {
            n232 = To Single Precision Float(number=w532) -> (single precision float=w534:sgl)
            n233 = Divide(x=w534, y=sgl 100.0) -> (x/y=w531:sgl)
          }
          frame True {
            n234 = To Single Precision Float(number=w537) -> (single precision float=w538:sgl)
            n235 = Divide(x=w538, y=sgl 100.0) -> (x/y=w535:sgl)
            n236 = Less Or Equal To 0?(x=w535) -> (x <= 0?=w536:bool)
            n237 = case shown="真" w536 {
              tunnel: [w541 sgl 0.015] -> w540
              tunnel: w535 -> [w541 _]
              frame False {
              }
              frame True {
              }
            }
          }
        }
        "COD浓度（mg/L)" <- w506
        n238 = To Single Precision Float(number=w524) -> (single precision float=w518:sgl)
        n239 = Build Array(w516, w515, w514) -> (w513:i16[])
        n240 = To Single Precision Float(number=w526) -> (single precision float=w523:sgl)
        n241 = To Single Precision Float(number=w525) -> (single precision float=w519:sgl)
        n242 = call "HexToDate.vi"("数组"=w513) -> ("DATE"=w517:timestamp[])  [unwired: 10 in]
        n243 = Number To Decimal String(number=w523) -> (decimal integer string=→"ORP-A":string)  [unwired: 1 in]
        n244 = Number To Decimal String(number=w519) -> (decimal integer string=→"ORP-B":string)  [unwired: 1 in]
        n245 = Number To Decimal String(number=w518) -> (decimal integer string=→"ORP-K":string)  [unwired: 1 in]
        n246 = Index Array(array=w517) -> (element=w511:timestamp)  [unwired: 1 in]
        n247 = Format Date/Time String(seconds (now)=w511) -> (date/time string=→"数据时间":string)  [unwired: 2 in]
      }
    }
    n248 = flat-sequence {
      frame #0 {
        # "测量状态显示"
        n249 = global read "COD内部交互全局.vi" "F0-F5"() -> (w414:u16[])
        n250 = global read "COD内部交互全局.vi" "测量状态"() -> (w422:u16[])
        n251 = To Single Precision Float(number=w414) -> (single precision float=w413:sgl[])
        n252 = Index Array(array=w413) -> (element #1=→"F0":sgl, element #2=→"F1":sgl, element #3=→"F2":sgl, element #4=→"F3":sgl, element #5=→"F4":sgl, element #6=→"F5":sgl)  [unwired: 6 in]
        n253 = To Word Integer(number=w422) -> (16bit integer=w432:i16[])
        n254 = Index Array(array=w432, index #1=0 ("索引"), index #4=3 ("索引"), index #14=13 ("索引"), index #15=14 ("索引"), index #21=20 ("索引"), index #32=31 ("索引")) -> (element #1=w436:i16, element #2=w435:i16, element #3=w434:i16, element #4=w418:i16, element #5=→"模式（受控）":i16, element #6=→"进样管":i16, element #7=→"高锰酸钾":i16, element #8=→"草酸钠":i16, element #9=→"硫酸":i16, element #10=w431:i16, element #11=w451:i16, element #12=w427:i16, element #13=→"报警数字":i16, element #14=w457:i16, element #15=w442:i16, element #16=→"多列列表框":i16, element #20=→"氢氧化钠":i16, element #21=w415:i16, element #33=→"分":i16, element #34=→"秒":i16)  [unwired: 28 in, 14 out]
        "CODMn工作状态" <- w418
        n255 = global write "COD内部交互全局.vi" "基本量程实时读取"(w415) -> ()
        n256 = Equal?(x=w418, y=T1."水样测试" ("CODMn工作状态")) -> (x = y?=w416:bool)
        n257 = Build Array(w436, w435, w434) -> (w437:i16[])
        n258 = To Single Precision Float(number=w431) -> (single precision float=→"实时ORP/光值":sgl)
        n259 = Number To Decimal String(number=w415) -> (decimal integer string=→"基本量程(显示)":string)  [unwired: 1 in]
        n260 = Equal?(x=w427, y=u16 1) -> (x = y?=→"排液标记":bool)
        n261 = Equal?(x=w427, y=u16 2) -> (x = y?=→"断电排液标记":bool)
        n262 = Divide(x=w451, y=u16 10) -> (x/y=→"消解温度℃":dbl)
        n263 = Divide(x=w457, y=u16 1000) -> (x/y=→"零点滴定值":dbl)
        n264 = Divide(x=w442, y=u16 1000) -> (x/y=→"标度滴定值":dbl)
        n265 = case shown="真" w416 {
          tunnel: w415 -> [_ w460]
          frame False {
          }
          frame True {
            n266 = global write "CODMn断电保存全局变量.vi" "水样测试量程"(w460) -> ()
          }
        }
        n267 = call "HexToDate.vi"("数组"=w437) -> ("DATE"=w433:timestamp[])  [unwired: 10 in]
        n268 = Index Array(array=w433) -> (element=→"仪器时间":timestamp)  [unwired: 1 in]
      }
    }
    n269 = flat-sequence {
      frame #0 {
        # "报警状态显示"
        n270 = global read "COD内部交互全局.vi" "报警点位"() -> (w475:bool[])
        n271 = Index Array(array=w475, index #1=0 ("索引")) -> (element #1=w472:bool, element #2=w471:bool, element #3=w470:bool, element #4=w469:bool, element #5=w468:bool, element #6=w467:bool, element #7=w466:bool, element #8=w465:bool, element #9=w464:bool, element #11=w463:bool, element #13=w462:bool, element #14=w461:bool)  [unwired: 13 in, 2 out]
        "ORP故障" <- w472
        "温控器故障" <- w471
        "加热故障" <- w464
        "高锰酸钾报警" <- w466
        "草酸钠报警" <- w465
        "测量错误" <- w470
        "校零错误" <- w469
        "校标错误" <- w468
        "进水样超量程" <- w467
        "排液故障" <- w463
        "60分钟超时报警" <- w462
        "进样无液体告警" <- w461
        n272 = Compound Arithmetic op=OR ("复合运算")(w472, w471, w464, w466, w465, w470, w468, w469, w467, w463, w462) -> (→"故障标记":bool)
        n273 = Bundle By Name(cluster=T13 {"ORP故障"=FALSE, "温控器故障"=FALSE, "加热故障"=FALSE, "高锰酸钾报警"=FALSE, "草酸钠报警"=FALSE, "测量错误"=FALSE, "校零错误"=FALSE, "校标错误"=FALSE, " 进水样超量程"=FALSE, "排液阀故障"=FALSE, "60分钟超时报警"=FALSE, "进样无液体报警"=FALSE} ("报警簇"), "ORP故障"=w472, "温控器故障"=w471, "加热故障"=w464, "高锰酸钾报警"=w466, "草酸钠报警"=w465, "测量错误"=w470, "校零错误"=w469, "校标错误"=w468, "进水样超量程"=w467, "排液阀故障"=w463, "60分钟超时报警"=w462, "进样无液体报警"=w461) -> (w473:T13)
        n274 = global write "COD内部交互全局.vi" "报警簇"(w473) -> ()
      }
    }
    n275 = flat-sequence {
      frame #0 {
        # "CODMn读取状态"
        n276 = global read "COD内部交互全局.vi" "温度"() -> (w505:bool[])
        n277 = global read "COD内部交互全局.vi" "M输出点"() -> (w504:bool[])
        n278 = Index Array(array=w505) -> (element=→"加热":bool)  [unwired: 1 in]
        n279 = Index Array(array=w504) -> (element #1=→"搅拌":bool, element #4=→"进水样":bool, element #5=→"进蒸馏水":bool, element #6=→"进标液":bool, element #7=→"进零点核查样":bool, element #8=→"进加标回收样":bool, element #9=→"进高锰酸钾":bool, element #10=→"进草酸钠":bool, element #11=→"进硫酸":bool)  [unwired: 11 in, 2 out]
      }
    }
    n280 = flat-sequence {
      frame #0 {
        # "工作状态显示"
        n281 = local read "CODMn工作状态"() -> (w373:T1)
        n282 = Not Equal To 0?(x=w373) -> (x != 0?=w372:bool)
        n283 = Equal?(x=w373, y=u16 0) -> (x = y?=→"待机":bool)
        n284 = Equal?(x=w373, y=u16 8) -> (x = y?=→"校零标记":bool)
        n285 = Equal?(x=w373, y=u16 1) -> (x = y?=→"水样测量":bool)
        n286 = Equal?(x=w373, y=u16 9) -> (x = y?=→"校标标记":bool)
        n287 = Equal?(x=w373, y=u16 7) -> (x = y?=→"质控样测量":bool)
        n288 = Equal?(x=w373, y=u16 5) -> (x = y?=→"空白测试标记":bool)
        n289 = Equal?(x=w373, y=u16 4) -> (x = y?=→"跨度核查标记":bool)
        n290 = Equal?(x=w373, y=u16 3) -> (x = y?=→"零点核查标记":bool)
        n291 = Equal?(x=w373, y=u16 2) -> (x = y?=→"标样核查标记":bool)
        n292 = Equal?(x=w373, y=u16 6) -> (x = y?=→"平行样测量":bool)
        n293 = Equal?(x=w373, y=u16 10) -> (x = y?=→"加标回收测量":bool)
        n294 = case shown="真" w372 {
          tunnel: w373 -> [_ w397]
          frame False {
          }
          frame True {
            n295 = case shown="\"水样测试\"" w397 {
              tunnel: [_ u16 0 ("y") u16 1 ("y") u16 2 ("y") u16 3 ("y") u16 4 ("y") u16 6 ("y") _ u16 7 ("y") u16 8 ("y") u16 5 ("y")] -> w396
              frame "空闲", Default {
              }
              frame "水样测试" {
              }
              frame "标样核查" {
              }
              frame "零点核查" {
              }
              frame "跨度核查" {
              }
              frame "空白测试" {
              }
              frame "平行样测试" {
              }
              frame "质控样" {
              }
              frame "空白校准" {
              }
              frame "标样校准" {
              }
              frame "加标回收" {
              }
            }
            n296 = global write "COD内部交互全局.vi" "测量模式数字"(w396) -> ()
          }
        }
      }
    }
    n297 = Get Date/Time In Seconds() -> (seconds since 1Jan1904=→"系统时间":timestamp)
    n298 = First Call?() -> (First Call?: T/F=w361:bool)
    n299 = Wait (ms)(milliseconds to wait=u32 1000 ("等待时间（毫秒）")) -> ()  [unwired: 1 out]
    n300 = case shown="真" w361 {
      tunnel: w363 -> [w479 w490]
      tunnel: w362 -> [w478 w489]
      tunnel: [w479 w481] -> w359
      tunnel: [w478 w480] -> w358
      frame False {
      }
      frame True {
        n301 = Bundle By Name(cluster=cluster{"命令":string} {"命令"=""} ("元素"), "命令"="CODMn读取参数" ("名称（未命名）")) -> (w493:cluster{"命令":string})
        n302 = Bundle By Name(cluster=cluster{"命令":string} {"命令"=""} ("元素"), "命令"="CODMn读取公式" ("名称（未命名）")) -> (w484:cluster{"命令":string})
        n303 = Enqueue Element(queue=w490, element=w493, timeout in ms (-1)=1000 ("超时毫秒(-1)"), error in (no error)=w489) -> (queue out=w483:refnum<queue>, error out=w482:errorcluster)  [unwired: 1 out]
        n304 = Enqueue Element(queue=w483, element=w484, timeout in ms (-1)=1000 ("超时毫秒(-1)"), error in (no error)=w482) -> (queue out=w481:refnum<queue>, error out=w480:errorcluster)  [unwired: 1 out]
      }
    }
    n305 = Get Queue Status(queue=w359, error in (no error)=w358) -> (queue out=w355:refnum<queue>, error out=w354:errorcluster, # elements in queue=w357:i32)  [unwired: 1 in, 5 out]
    n306 = Equal To 0?(x=w357) -> (x = 0?=w356:bool)
    n307 = case shown="真" w356 {
      tunnel: w355 -> [_ w367]
      tunnel: w354 -> [_ w366]
      frame False {
      }
      frame True {
        n308 = Bundle By Name(cluster=cluster{"命令":string} {"命令"=""} ("元素"), "命令"="CODMn读取" ("名称（未命名）")) -> (w369:cluster{"命令":string})
        n309 = Enqueue Element(queue=w367, element=w369, timeout in ms (-1)=1000 ("超时毫秒(-1)"), error in (no error)=w366) -> ()  [unwired: 3 out]
      }
    }
  }
  n310 = while {
    tunnel: w29 -> [w546]
    tunnel: w28 -> [w545]
    tunnel: w11 -> [w544]
    tunnel: w6 -> [w543]
    stop <- FALSE stop-if-true
    # "主线事件"
    n311 = event shown="[19] \"温度补偿\": 值改变" {
      selector: _ -> [_ _ _ _ _ _ _ _ _ _ _ _ _ _ _ _ _ _ _ _ _]
      dyn-events: _ -> [_ _ _ _ _ _ _ _ _ _ _ _ _ _ _ _ _ _ _ _ _]
      timeout: _ -> [_ _ _ _ _ _ _ _ _ _ _ _ _ _ _ _ _ _ _ _ _]
      tunnel: w546 -> [_ _ _ _ w625 _ _ w668 _ _ _ _ _ _ _ w723 w730 w752 w796 w813 _]
      tunnel: w545 -> [_ _ _ _ w624 _ _ w667 _ _ _ _ _ _ _ w722 w729 w751 w795 w812 _]
      tunnel: w544 -> [_ _ _ _ _ _ _ w666 _ _ _ _ _ _ _ _ _ _ _ _ _]
      tunnel: w543 -> [_ _ _ _ w620 _ _ _ _ _ _ _ _ _ _ _ _ _ _ _ _]
      event "单步启动": Value Change {
        n312 = event-data() -> ()  [unwired: 1 in, 6 out]
        n313 = call "CODMn手动控制框.vi"() -> ()  [unwired: 12 in]
      }
      event "启动": Mouse Down {
        n314 = event-data() -> ()  [unwired: 1 in, 8 out]
        n315 = global read "COD内部交互全局.vi" "基本量程实时读取"() -> (w550:enum16{"L", "H", "AUTO"})
        n316 = call "启动测量模式选择对话框.vi"("量程选择"=w550) -> ("标样浓度输出"=w548:dbl, "量程选择输出"=w549:enum16{"L", "H", "AUTO"}, "启动选择输出"=w554:u16)  [unwired: 8 in]
        n317 = Not Equal?(x=w554, y=u16 7) -> (x != y?=w552:bool)
        n318 = Not Equal?(x=w554, y=u16 8) -> (x != y?=w551:bool)
        n319 = And(x=w552, y=w551) -> (x .and. y?=w556:bool)
        n320 = case shown="真" w556 {
          tunnel: w554 -> [_ w571]
          tunnel: w549 -> [_ w562]
          tunnel: w548 -> [_ w561]
          frame False {
            n321 = One Button Dialog(message="请到校准配置里面进行校准操作！" ("消息")) -> ()  [unwired: 1 in, 1 out]
          }
          frame True {
            n322 = case shown="4" w571 {
              tunnel: [u16 4608 ("address") u16 4608 ("address") u16 4608 ("address") u16 4608 ("address") u16 4608 ("address") u16 4608 ("address") u16 4608 ("address") u16 4608 ("address") u16 4608 ("address") u16 4608 ("address")] -> w564
              tunnel: [u16 1 ("address") u16 2 ("address") u16 3 ("address") u16 4 ("address") u16 5 ("address") u16 7 ("address") u16 6 ("address") u16 8 ("address") u16 9 ("address") u16 0 ("address")] -> w568
              tunnel: w561 -> [_ _ _ _ _ _ _ _ _ _]
              frame 0 {
              }
              frame 1 {
              }
              frame 2 {
              }
              frame 3 {
              }
              frame 4 {
              }
              frame 5 {
              }
              frame 6 {
              }
              frame 7 {
              }
              frame 8 {
              }
              frame 9, Default {
              }
            }
            n323 = case shown="\"H\"" w562 {
              tunnel: [w572 w576 errorcluster {"status"=FALSE, "code"=0, "source"=""} ("error out")] -> w560
              frame "L", Default {
                n324 = call "CODMnMB_api.vi"("STEP"=enum16{"open", "read", "write", "close"}."write", "values"=u16[] [0], "starting address"=u16 4276) -> ("error out"=w572:errorcluster)  [unwired: 6 in, 2 out]
              }
              frame "H" {
                n325 = call "CODMnMB_api.vi"("STEP"=enum16{"open", "read", "write", "close"}."write", "values"=u16[] [1], "starting address"=u16 4276) -> ("error out"=w576:errorcluster)  [unwired: 6 in, 2 out]
              }
              frame "AUTO" {
              }
            }
            n326 = Not Equal?(x=w571, y=u16 9) -> (x != y?=w566:bool)
            n327 = global write "CODMN外部API.vi" "手动启动CODMn"(w566) -> ()
            n328 = call "单步测试一键复位.vi"("Error in"=w560) -> ("error out"=w559:errorcluster)  [unwired: 10 in]
            n329 = call <vilib>:"Clear Errors.vi"("error in (no error)"=w559) -> ("error out"=w558:errorcluster)  [unwired: 5 in, 1 out]
            n330 = Insert Into Array(array=u16[] [] ("values"), index=0 ("索引"), new element=w568) -> (w563:u16[])
            n331 = call "CODMnMB_api.vi"("STEP"=enum16{"open", "read", "write", "close"}."write", "Error in"=w558, "values"=w563, "starting address"=w564) -> ()  [unwired: 5 in, 3 out]
          }
        }
      }
      event "停止": Value Change {
        n332 = event-data() -> ()  [unwired: 1 in, 6 out]
        n333 = Two Button Dialog(message="确认是否停止？" ("消息"), 1:"否" ("F按钮名称（“取消”）"), 2:"是" ("T按钮名称（“确定”）")) -> (T button?=w603:bool)
        n334 = case shown="真" w603 {
          frame False {
          }
          frame True {
            n335 = Obtain Notifier(name (unnamed)="CODMn" ("名称（未命名）"), notification data type=FALSE) -> (notifier out=w609:refnum<notifier>, error out=w607:errorcluster)  [unwired: 2 in, 1 out]
            n336 = Send Notification(notification=TRUE ("通知"), notifier=w609, error in (no error)=w607) -> (notifier out=w606:refnum<notifier>, error out=w605:errorcluster)
            n337 = call "CODMnMB_api.vi"("STEP"=enum16{"open", "read", "write", "close"}."write", "values"=u16[] [11], "starting address"=u16 4608) -> ()  [unwired: 6 in, 3 out]
            n338 = Release Notifier(notifier=w606, error in (no error)=w605) -> ()  [unwired: 1 in, 3 out]
          }
        }
      }
      event "手动控制": Value Change {
        n339 = event-data() -> ()  [unwired: 1 in, 6 out]
        n340 = call "数字密码键盘.vi"() -> ("NewNumber"=w615:u32)  [unwired: 1 in]
        n341 = Equal?(x=w615, y=8.0) -> (x = y?=w616:bool)
        n342 = case shown="假" w616 {
          frame False {
            n343 = call "窗口弹出对话框(子VI).vi"("消息"="密码错误") -> ()  [unwired: 10 in, 1 out]
          }
          frame True {
          }
        }
      }
      event "参数配置": Value Change {
        (unwired) u16 20 ("number of holding registers")
        n344 = event-data() -> ()  [unwired: 1 in, 6 out]
        n345 = global read "CODMN外部API.vi" "ping"() -> (w623:bool)
        n346 = invoke on="子面板" class="SubPnl" method="Remove VI"() -> (error out=w619:errorcluster)  [unwired: 3 in, 2 out]
        n347 = property on="窗格" class="Pane"("Origin"=T2 {"Horizontal"=0, "Vertical"=650} ("原点")) -> ()  [unwired: 2 in, 2 out]
        n348 = case shown="假" w623 {
          tunnel: [w635 w638] -> w622
          frame False {
            n349 = global read "COD内部交互全局.vi" "配置文件ini"() -> (w637:string)
            n350 = call <vilib>:"Application Directory.vi"() -> ("Application Directory"=w636:path)
            n351 = Build Path(base path=w636, name or relative path=w637) -> (appended path=w635:path)
          }
          frame True {
            n352 = global read "CODMN外部API.vi" "配置文件 path"() -> (w638:path)
          }
        }
        n353 = invoke on="子面板" class="SubPnl" method="Insert VI"(error in=w619, "VI Ref"=w620) -> ()  [unwired: 2 in, 4 out]
        n354 = Bundle By Name(cluster=cluster{"命令":string} {"命令"=""} ("元素"), "命令"="CODMn读取参数" ("名称（未命名）")) -> (w626:cluster{"命令":string})
        n355 = Enqueue Element(queue=w625, element=w626, error in (no error)=w624) -> ()  [unwired: 1 in, 3 out]
        n356 = call <vilib>:"Open Config Data.vi"("configuration file path"=w622) -> ("error out"=w632:errorcluster, "refnum"=w629:T4)  [unwired: 8 in, 1 out]
        n357 = vi-ref "斯坦道CODMn.lvlib:CODMn断电保存全局变量.vi"() -> (w630:refnum<vi>)
        n358 = call <userlib>:"Read Panel from INI__ogtk.vi"("error in (no error)"=w632, "VI ref"=w630, "refnum"=w629) -> ("error out"=w633:errorcluster, "refnum out"=w631:T4)  [unwired: 7 in]
        n359 = call <vilib>:"Close Config Data.vi"("error in (no error)"=w633, "refnum"=w631) -> ("error out"=w621:errorcluster)  [unwired: 8 in, 1 out]
        n360 = call <vilib>:"Clear Errors.vi"("error in (no error)"=w621) -> ()  [unwired: 5 in, 2 out]
      }
      event "布尔": Value Change {
        n361 = event-data() -> ("CtlRef"=w639:refnum<vi>, "NewVal"=w640:bool)  [unwired: 1 in, 4 out]
        n362 = case shown="真" w640 {
          tunnel: w639 -> [_ w643]
          frame False {
            n363 = global write "CODMN外部API.vi" "权限等级"(enum16{"一级权限", "二级权限", "三级权限", "超级权限"}."一级权限" ("权限等级")) -> ()
          }
          frame True {
            n364 = property class="Bool (严格)"(reference=w643, "Value"=FALSE ("值")) -> ()  [unwired: 1 in, 2 out]
            n365 = global read "CODMN外部API.vi" "权限密码"() -> (w644:u32[])
            n366 = global read "CODMN外部API.vi" "权限等级"() -> (w646:enum16{"一级权限", "二级权限", "三级权限", "超级权限"})
            n367 = call "密码权限设置.vi"("权限输入"=w646, "权限密码"=w644) -> ("权限输出"=w645:enum16{"一级权限", "二级权限", "三级权限", "超级权限"})  [unwired: 9 in]
            n368 = global write "CODMN外部API.vi" "权限等级"(w645) -> ()
          }
        }
      }
      event "保存": Value Change {
        n369 = event-data() -> ()  [unwired: 1 in, 6 out]
        n370 = local read "通讯状态"() -> (w647:bool)
        n371 = Two Button Dialog(message="确定保存参数，保存参数将会替换原有参数！" ("消息")) -> (T button?=w649:bool)  [unwired: 2 in]
        n372 = case shown="真" w649 {
          tunnel: w647 -> [_ w650]
          frame False {
          }
          frame True {
            n373 = case shown="真" w650 {
              frame False {
                n374 = One Button Dialog(message="保存失败，当前无通讯！" ("消息")) -> ()  [unwired: 1 in, 1 out]
              }
              frame True {
                n375 = global read "COD内部交互全局.vi" "保存参数"() -> (w652:dbl[])
                n376 = One Button Dialog(message="参数保存成功！" ("消息")) -> ()  [unwired: 1 in, 1 out]
                n377 = global read "COD内部交互全局.vi" "采水泵参数"() -> (w653:i32[])
                n378 = call "CODMnMB_api.vi"("STEP"=enum16{"open", "read", "write", "close"}."write", "values"=w652, "starting address"=u16 4272) -> ("error out"=w660:errorcluster)  [unwired: 6 in, 2 out]
                n379 = call "CODMnMB_api.vi"("STEP"=enum16{"open", "read", "write", "close"}."write", "Error in"=w660, "values"=w653, "starting address"=u16 5596) -> ("error out"=w657:errorcluster)  [unwired: 5 in, 2 out]
                n380 = global read "COD内部交互全局.vi" "泵校准参数"() -> (w654:T14)
                n381 = call <vilib>:"Clear Errors.vi"("error in (no error)"=w657) -> ("error out"=w655:errorcluster)  [unwired: 5 in, 1 out]
                n382 = call "PLC版CODMn泵校准数据插入.vi"("data"=w654, "错误输入（无错误）"=w655) -> ("错误输出"=w656:errorcluster)  [unwired: 8 in]
                n383 = flat-sequence {
                  tunnel: w656 -> [_]
                  frame #0 {
                    n384 = global write "COD内部交互全局.vi" "更换泵管"(FALSE ("更换泵管")) -> ()
                  }
                }
              }
            }
          }
        }
      }
      event "校准配置": Value Change {
        n385 = event-data() -> ()  [unwired: 1 in, 6 out]
        n386 = invoke on="子面板" class="SubPnl" method="Remove VI"() -> (error out=w665:errorcluster)  [unwired: 3 in, 2 out]
        n387 = property on="窗格" class="Pane"("Origin"=T2 {"Horizontal"=0, "Vertical"=1300} ("原点")) -> ()  [unwired: 2 in, 2 out]
        n388 = invoke on="子面板" class="SubPnl" method="Insert VI"(error in=w665, "VI Ref"=w666) -> ()  [unwired: 2 in, 4 out]
        n389 = Bundle By Name(cluster=cluster{"命令":string} {"命令"=""} ("元素"), "命令"="CODMn读取公式" ("名称（未命名）")) -> (w669:cluster{"命令":string})
        n390 = Enqueue Element(queue=w668, element=w669, error in (no error)=w667) -> ()  [unwired: 1 in, 3 out]
      }
      event "返回": Value Change {
        n391 = event-data() -> ()  [unwired: 1 in, 6 out]
        n392 = property on="窗格" class="Pane"("Origin"=T2 {"Horizontal"=0, "Vertical"=0} ("原点")) -> ()  [unwired: 2 in, 2 out]
      }
      event "关闭": Value Change {
        n393 = event-data() -> ()  [unwired: 1 in, 6 out]
        n394 = property on="窗格" class="Pane"("Origin"=T2 {"Horizontal"=0, "Vertical"=0} ("原点")) -> ()  [unwired: 2 in, 2 out]
      }
      event Application Instance Close {
        n395 = event-data() -> ()  [unwired: 1 in, 4 out]
      }
      event "时间校准": Value Change {
        n396 = event-data() -> ()  [unwired: 1 in, 6 out]
        n397 = Get Date/Time In Seconds() -> (seconds since 1Jan1904=w683:timestamp)
        n398 = Build Array(w683) -> (w682:timestamp[])
        n399 = call "DateToHex.vi"("DATE"=w682) -> ("数组"=w680:u16[])  [unwired: 10 in]
        n400 = Insert Into Array(array=u16[] [1] ("values"), index=1 ("索引"), new element=w680) -> (w676:u16[])
        n401 = call "CODMnMB_api.vi"("STEP"=enum16{"open", "read", "write", "close"}."write", "values"=w676, "starting address"=u16 4612) -> ("error out"=w675:errorcluster)  [unwired: 6 in, 2 out]
        n402 = call <vilib>:"Clear Errors.vi"("error in (no error)"=w675) -> ()  [unwired: 5 in, 2 out]
      }
      event "故障清除": Value Change {
        n403 = event-data() -> ()  [unwired: 1 in, 6 out]
        n404 = call "CODMnMB_api.vi"("STEP"=enum16{"open", "read", "write", "close"}."write", "values"=u16[] [1], "starting address"=u16 4611) -> ()  [unwired: 6 in, 3 out]
      }
      event "仪器参数": Value Change {
        n405 = event-data() -> ()  [unwired: 1 in, 6 out]
        n406 = global read "CODMn断电保存全局变量.vi" "CODMn仪器参数"() -> (w687:T6)
        n407 = call "仪器参数设置.vi"("氨氮仪器参数"=w687) -> ("仪器参数设置输出"=w688:T15)  [unwired: 10 in]
        n408 = Unbundle By Name(w688) -> ("确定"=w689:bool)
        n409 = case shown="真" w689 {
          tunnel: w688 -> [_ w691]
          tunnel: w687 -> [_ w690]
          frame False {
          }
          frame True {
            n410 = flat-sequence {
              tunnel: w691 -> [w710]
              tunnel: w690 -> [w709]
              frame #0 {
                n411 = Unbundle By Name(w710) -> ("测量量程"=w708:dbl, "测量精度"=w707:dbl, "测量间隔"=w693:dbl, "消解温度"=w706:dbl, "消解时长"=w705:dbl, "空白校准时间"=w704:timestamp, "曲线截距"=w703:dbl, "曲线斜率"=w702:dbl, "测量检出限"=w701:dbl, "测量信号值"=w700:dbl, "线性相关系数"=w699:dbl, "二次多项式系数"=w698:dbl, "标样校准时间"=w697:timestamp, "稀释倍数"=w696:dbl)
                n412 = Bundle By Name(cluster=w709, "测量量程"=w708, "测量精度"=w707, "测量间隔"=w693, "消解温度"=w706, "消解时长"=w705, "空白校准时间"=w704, "曲线截距"=w703, "曲线斜率"=w702, "测量检出限"=w701, "测量信号值"=w700, "线性相关系数"=w699, "二次多项式系数"=w698, "标样校准时间"=w697, "稀释倍数"=w696) -> (w695:T6)
                n413 = global read "CODMn断电保存全局变量.vi" "运行周期"() -> (w694:T5)
                n414 = Bundle By Name(cluster=w694, "测量间隔"=w693) -> (w692:T5)
                n415 = global write "CODMn断电保存全局变量.vi" "CODMn仪器参数"(w695) -> ()
                n416 = global write "CODMn断电保存全局变量.vi" "运行周期"(w692) -> ()
              }
              frame #1 {
                n417 = call "配置文件保存.vi"() -> ()  [unwired: 12 in]
                n418 = global write "CODMn断电保存全局变量.vi" "关键参数改变"(TRUE ("校准信息改变")) -> ()
              }
            }
          }
        }
      }
      event "查看曲线": Value Change {
        n419 = event-data() -> ()  [unwired: 1 in, 6 out]
        n420 = vi-ref "斯坦道CODMn.lvlib:读取CODMn数据波形新.vi"() -> (w713:refnum<vi>)
        n421 = property class="VI"(reference=w713) -> ("Name"=w719:string)  [unwired: 1 in, 2 out]
        n422 = Open VI Reference(type specifier VI Refnum (for type only)=refnum<vi> refnum, vi path=w719, options=128 ("选项")) -> (vi reference=w717:refnum<vi>, error out=w716:errorcluster)  [unwired: 3 in]
        n423 = call-by-ref "?"(reference=w717, error in=w716) -> (reference out=w714:refnum<vi>, error out=w715:errorcluster)  [unwired: 12 in]
        n424 = Close Reference(reference=w714, error in (no error)=w715) -> ()  [unwired: 1 out]
      }
      event "释放串口": Value Change {
        n425 = event-data() -> ()  [unwired: 1 in, 6 out]
        n426 = Two Button Dialog(message="确认是否释放串口，释放串口将导致通信失败！" ("消息")) -> (T button?=w720:bool)  [unwired: 2 in]
        n427 = case shown="真" w720 {
          tunnel: w723 -> [_ w725]
          tunnel: w722 -> [_ w724]
          frame False {
          }
          frame True {
            n428 = Bundle By Name(cluster=cluster{"命令":string} {"命令"=""} ("元素"), "命令"="停用模块" ("名称（未命名）")) -> (w726:cluster{"命令":string})
            n429 = Enqueue Element(queue=w725, element=w726, error in (no error)=w724) -> ()  [unwired: 1 in, 3 out]
          }
        }
      }
      event "打开串口": Value Change {
        n430 = event-data() -> ()  [unwired: 1 in, 6 out]
        n431 = flat-sequence {
          tunnel: w730 -> [w738]
          tunnel: w729 -> [w737]
          frame #0 {
            n432 = global read "CODMn断电保存全局变量.vi" "VISA resource name"() -> (w741:refnum<visa-resource-name>)
            n433 = global read "CODMn断电保存全局变量.vi" "MB通信方式选择"() -> (w734:enum16{"串口", "TCP"})
            n434 = global read "CODMn断电保存全局变量.vi" "PORT"() -> (w732:string)
            n435 = global read "CODMn断电保存全局变量.vi" "IP"() -> (w733:string)
            n436 = call "串口配置.vi"("PORT"=w732, "IP"=w733, "MB通信方式选择"=w734, "请选择串口:"=w741) -> ("PORT 2"=w735:string, "IP 2"=w736:string, "确认 2"=w739:bool, "VISA资源名称 2"=w740:refnum<visa-resource-name>, "MB通信方式选择 2"=w731:enum16{"串口", "TCP"})  [unwired: 3 in]
            n437 = case shown="真" w739 {
              tunnel: w740 -> [_ w750]
              tunnel: w738 -> [_ w746]
              tunnel: w737 -> [_ w745]
              tunnel: w736 -> [_ w744]
              tunnel: w735 -> [_ w743]
              tunnel: w731 -> [_ w742]
              frame False {
              }
              frame True {
                n438 = global write "CODMn断电保存全局变量.vi" "IP"(w744) -> ()
                n439 = global write "CODMn断电保存全局变量.vi" "PORT"(w743) -> ()
                n440 = global write "CODMn断电保存全局变量.vi" "VISA resource name"(w750) -> ()
                n441 = global write "CODMn断电保存全局变量.vi" "MB通信方式选择"(w742) -> ()
                n442 = Bundle By Name(cluster=cluster{"命令":string} {"命令"=""} ("元素"), "命令"="启用模块" ("名称（未命名）")) -> (w747:cluster{"命令":string})
                n443 = Enqueue Element(queue=w746, element=w747, error in (no error)=w745) -> ()  [unwired: 1 in, 3 out]
              }
            }
          }
          frame #1 {
            n444 = call "配置文件保存.vi"() -> ()  [unwired: 12 in]
          }
        }
      }
      event "更新程序": Value Change {
        n445 = event-data() -> ("CtlRef"=w753:refnum<vi>, "NewVal"=w754:bool)  [unwired: 1 in, 4 out]
        n446 = case shown="真" w754 {
          tunnel: w753 -> [_ w763]
          tunnel: w752 -> [w756 w762]
          tunnel: w751 -> [w755 w761]
          frame False {
            n447 = Bundle By Name(cluster=cluster{"命令":string} {"命令"=""} ("元素"), "命令"="启用模块" ("名称（未命名）")) -> (w757:cluster{"命令":string})
            n448 = Enqueue Element(queue=w756, element=w757, error in (no error)=w755) -> ()  [unwired: 1 in, 3 out]
          }
          frame True {
            n449 = Two Button Dialog(message="警告，非专业人士请勿进行此操作！！！\n请确认是否继续？" ("消息")) -> (T button?=w765:bool)  [unwired: 2 in]
            n450 = case shown="真" w765 {
              tunnel: w763 -> [w781 _]
              tunnel: w762 -> [_ w789]
              tunnel: w761 -> [_ w788]
              tunnel: [errorcluster {"status"=TRUE, "code"=0, "source"=""} ("error out") w782] -> w760
              frame False {
                n451 = property class="Bool (严格)"(reference=w781, "Value"=FALSE ("释放串口")) -> ()  [unwired: 1 in, 2 out]
              }
              frame True {
                n452 = Bundle By Name(cluster=cluster{"命令":string} {"命令"=""} ("元素"), "命令"="CODMn程序更新" ("名称（未命名）")) -> (w792:cluster{"命令":string})
                n453 = Bundle By Name(cluster=cluster{"命令":string} {"命令"=""} ("元素"), "命令"="停用模块" ("名称（未命名）")) -> (w783:cluster{"命令":string})
                n454 = Enqueue Element(queue=w789, element=w792, error in (no error)=w788) -> (queue out=w787:refnum<queue>, error out=w786:errorcluster)  [unwired: 1 in, 1 out]
                n455 = Enqueue Element(queue=w787, element=w783, error in (no error)=w786) -> (error out=w782:errorcluster)  [unwired: 1 in, 2 out]
              }
            }
            n456 = case shown="无错误" w760 {
              frame No Error {
                n457 = call "文件对话框"("start path"=path "D:/SRC") -> ("selected path"=w768:path, "cancelled"=w766:bool)  [unwired: 11 in, 2 out]
                n458 = case shown="假" w766 {
                  tunnel: w768 -> [w773 _]
                  frame False {
                    n459 = Path To String(path=w773) -> (string=w770:string)
                    n460 = Format Into String(format string="  - \"%s\"" ("格式字符串"), initial string="\"C:\\Program Files\\Fatek\\WinProladder\\WProlad.exe\"" ("command line"), w770) -> (resulting string=w771:string)  [unwired: 1 in, 1 out]
                    n461 = call <vilib>:"System Exec.vi"("command line"=w771) -> ("error out"=w774:errorcluster)  [unwired: 7 in, 3 out]
                    n462 = case shown="错误" w774 {
                      tunnel: w770 -> [_ w777]
                      frame No Error {
                      }
                      frame Error {
                        n463 = Format Into String(format string="  - \"%s\"" ("格式字符串"), initial string="\"C:\\Program Files (x86)\\Fatek\\WinProladder\\WProlad.exe\"" ("command line"), w777) -> (resulting string=w775:string)  [unwired: 1 in, 1 out]
                        n464 = call <vilib>:"System Exec.vi"("command line"=w775) -> ()  [unwired: 7 in, 4 out]
                      }
                    }
                  }
                  frame True {
                  }
                }
              }
              frame Error {
              }
            }
          }
        }
      }
      event "序列号变更": Value Change {
        n465 = event-data() -> ()  [unwired: 1 in, 6 out]
        n466 = global read "COD内部交互全局.vi" "序列号:"() -> (w793:string)
        n467 = call "序列号写入.vi"("序列号:"=w793) -> ("确认 2"=w794:bool, "序列号输出"=w797:string)  [unwired: 9 in]
        n468 = case shown="真" w794 {
          tunnel: w797 -> [_ w803]
          tunnel: w796 -> [_ w799]
          tunnel: w795 -> [_ w798]
          frame False {
          }
          frame True {
            n469 = global write "COD内部交互全局.vi" "序列号:"(w803) -> ()
            n470 = Bundle By Name(cluster=cluster{"命令":string} {"命令"=""} ("元素"), "命令"="CODMn序列号写入" ("名称（未命名）")) -> (w800:cluster{"命令":string})
            n471 = Enqueue Element(queue=w799, element=w800, error in (no error)=w798) -> ()  [unwired: 1 in, 3 out]
          }
        }
      }
      event "温度补偿": Value Change {
        n472 = event-data() -> ()  [unwired: 1 in, 6 out]
        n473 = Bundle By Name(cluster=cluster{"命令":string} {"命令"=""} ("元素"), "命令"="CODMn读取参数" ("名称（未命名）")) -> (w814:cluster{"命令":string})
        n474 = vi-ref "斯坦道CODMn.lvlib:温度补偿.vi"() -> (w805:refnum<vi>)
        n475 = Enqueue Element(queue=w813, element=w814, error in (no error)=w812) -> ()  [unwired: 1 in, 3 out]
        n476 = property class="VI"(reference=w805) -> ("Name"=w811:string)  [unwired: 1 in, 2 out]
        n477 = Open VI Reference(type specifier VI Refnum (for type only)=refnum<vi> refnum, vi path=w811, options=128 ("选项")) -> (vi reference=w809:refnum<vi>, error out=w808:errorcluster)  [unwired: 3 in]
        n478 = call-by-ref "?"(reference=w809, error in=w808) -> (reference out=w806:refnum<vi>, error out=w807:errorcluster)  [unwired: 12 in]
        n479 = Close Reference(reference=w806, error in (no error)=w807) -> ()  [unwired: 1 out]
      }
      event Timeout {
        n480 = event-data() -> ()  [unwired: 1 in, 3 out]
      }
    }
  }
  n481 = property class="VI"(reference=w20, error in=w17) -> ("Name"=w21:string)  [unwired: 2 out]
  n482 = Open VI Reference(type specifier VI Refnum (for type only)=refnum<vi> refnum, vi path=w21, options=128 ("选项")) -> (vi reference=w23:refnum<vi>, error out=w25:errorcluster)  [unwired: 3 in]
  n483 = call-by-ref "?"(reference=w23, error in=w25) -> (reference out=w27:refnum<vi>, error out=w26:errorcluster)  [unwired: 12 in]
  n484 = Close Reference(reference=w27, error in (no error)=w26) -> ()  [unwired: 1 out]
